vi "Set DC Params.vi"(8 "error in (no error)":errorcluster, 10 "Step In":refnum<k7>, 11 "Power Sweep in":refnum<class "Power Sweep.lvclass">) -> (0 "error out":errorcluster, 2 "Step Out":refnum<k7>, 3 "Power Sweep out":refnum<class "Power Sweep.lvclass">)   [LabVIEW 2018, in "Power Sweep.lvlib" / "Power Sweep.lvclass"]
uses:
  Power Sweep.lvclass
  Power Sweep.lvclass/Power Sweep.ctl
  Read PAE Pins.vi
  Read PAE Enable Override.vi
  Read DC Pins.vi
  Plugins/TestStand API Tools (TSAT).lvlibp/Step Actions/TSAT Step Actions.lvlib
  Plugins/Measurement Interface.lvlibp/Measurement Interface.lvclass
  C:/Sequence Automation/Plugins/Measurement Interface.lvlibp/Measurement Interface.lvclass
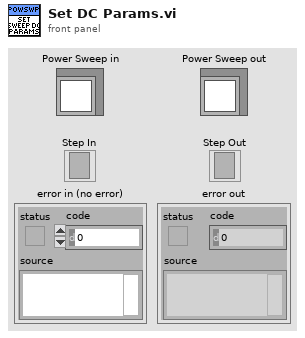
[diagram p1: front panel]
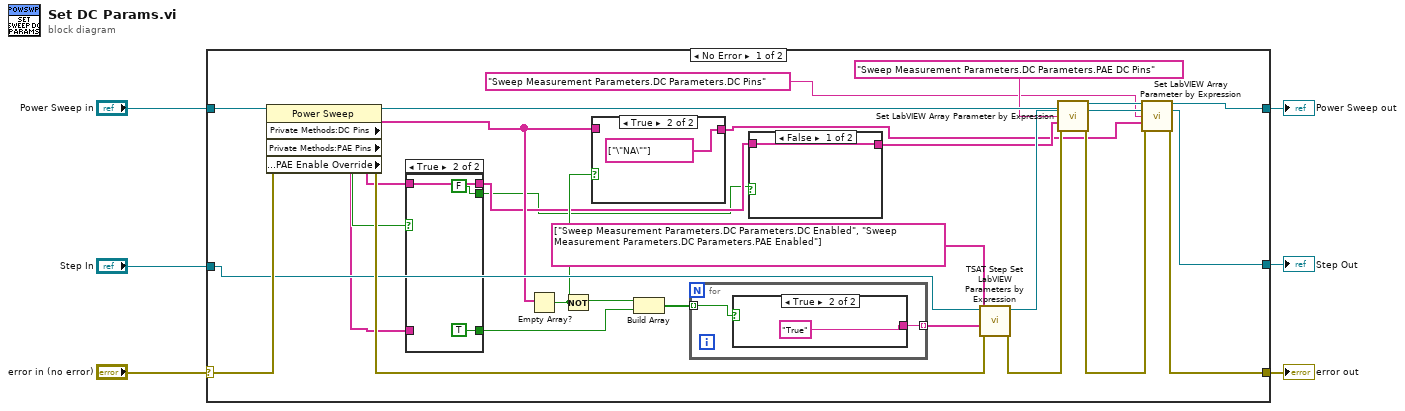
[diagram p0: block diagram]
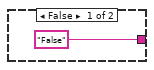
[diagram p2: hidden frame]
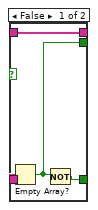
[diagram p3: hidden frame]
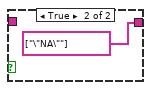
[diagram p4: hidden frame]
diagram:
  n1 = case shown="No Error" "error in (no error)" {
    selector: "error in (no error)" -> [w34 w51]
    tunnel: [w31 w51] -> w5
    tunnel: [w26 w50] -> w3
    tunnel: "Power Sweep in" -> [w33 w50]
    tunnel: "Step In" -> [w23 w49]
    tunnel: [w29 w49] -> w1
    frame No Error {
      n2 = property class="Power Sweep"(reference=w33, error in=w34) -> (reference out=w28:refnum<class "Power Sweep.lvclass">, error out=w25:errorcluster, "Private Methods:DC Pins"=w19:string[], "Private Methods:PAE Pins"=w18:string[], "Private Methods:PAE Enable Override"=w20:bool)
      n3 = case shown="True" w20 {
        tunnel: w19 -> [_ w44]
        tunnel: w18 -> [w40 _]
        tunnel: [w41 TRUE] -> w17
        tunnel: [w40 w44] -> w12
        tunnel: [w39 FALSE ("empty?")] -> w11
        frame False {
          n4 = Empty Array?(array=w40) -> (empty?=w39:bool)
          n5 = Not(x=w39) -> (.not. x?=w41:bool)
        }
        frame True {
        }
      }
      n6 = Empty Array?(array=w19) -> (empty?=w21:bool)
      n7 = Not(x=w21) -> (.not. x?=w13:bool)
      n8 = case shown="True" w21 {
        tunnel: w19 -> [w47 _]
        tunnel: [w47 string[] ["\"NA\""] ("Protected Methods:DC Pins")] -> w7
        frame False {
        }
        frame True {
        }
      }
      n9 = Build Array(w13, w17) -> (w16:bool[])
      n10 = for {
        tunnel: w16 -> [w36] mode=indexing
        tunnel: [w35] -> w15 mode=indexing
        n11 = case shown="True" w36 {
          tunnel: ["False" "True"] -> w35
          frame False {
          }
          frame True {
          }
        }
      }
      n12 = case shown="False" w11 {
        tunnel: w12 -> [w45 _]
        tunnel: [w45 string[] ["\"NA\""] ("Protected Methods:DC Pins")] -> w10
        frame False {
        }
        frame True {
        }
      }
      n13 = call "TSAT Step Set LabVIEW Parameters by Expression.vi"("Error In"=w25, "Value Expressions"=w15, "Parameters to Set"=string[] ["Sweep Measurement Parameters.DC Parameters.DC Enabled", "Sweep Measurement Parameters.DC Parameters.PAE Enabled"], "Step In"=w23) -> ("Error Out"=w24:errorcluster, "Step Out"=w22:refnum<k7>)  [unwired: 6 in]
      n14 = call "Set LabVIEW Array Parameter by Expression.vi"("Measurement Interface in"=w28, "Step In"=w22, "LabVIEW Parameter to Set"="Sweep Measurement Parameters.DC Parameters.PAE DC Pins", "Array of Expresssions"=w10, "error in (no error)"=w24) -> ("Measurement Interface out"=w27:refnum<class "Power Sweep.lvclass">, "Step Out"=w30:refnum<k7>, "error out"=w32:errorcluster)  [unwired: 8 in]
      n15 = call "Set LabVIEW Array Parameter by Expression.vi"("Measurement Interface in"=w27, "Step In"=w30, "LabVIEW Parameter to Set"="Sweep Measurement Parameters.DC Parameters.DC Pins", "Array of Expresssions"=w7, "error in (no error)"=w32) -> ("Measurement Interface out"=w26:refnum<class "Power Sweep.lvclass">, "Step Out"=w29:refnum<k7>, "error out"=w31:errorcluster)  [unwired: 8 in]
    }
    frame Error {
    }
  }
  "error out" <- w5
  "Power Sweep out" <- w3
  "Step Out" <- w1
